vi "Properties_Insert Dotted Properties.vi"(11 "Property Info Array In":T1(array[cluster])) -> (1 "exe time (ms)":u32, 2 "Stop":bool, 3 "Property Info Array Out":T1(array[cluster]))   [LabVIEW 2023]
doc: "Find all dottable properties and insert dotted properties after them in list."
panel:
  out "dotted":i32
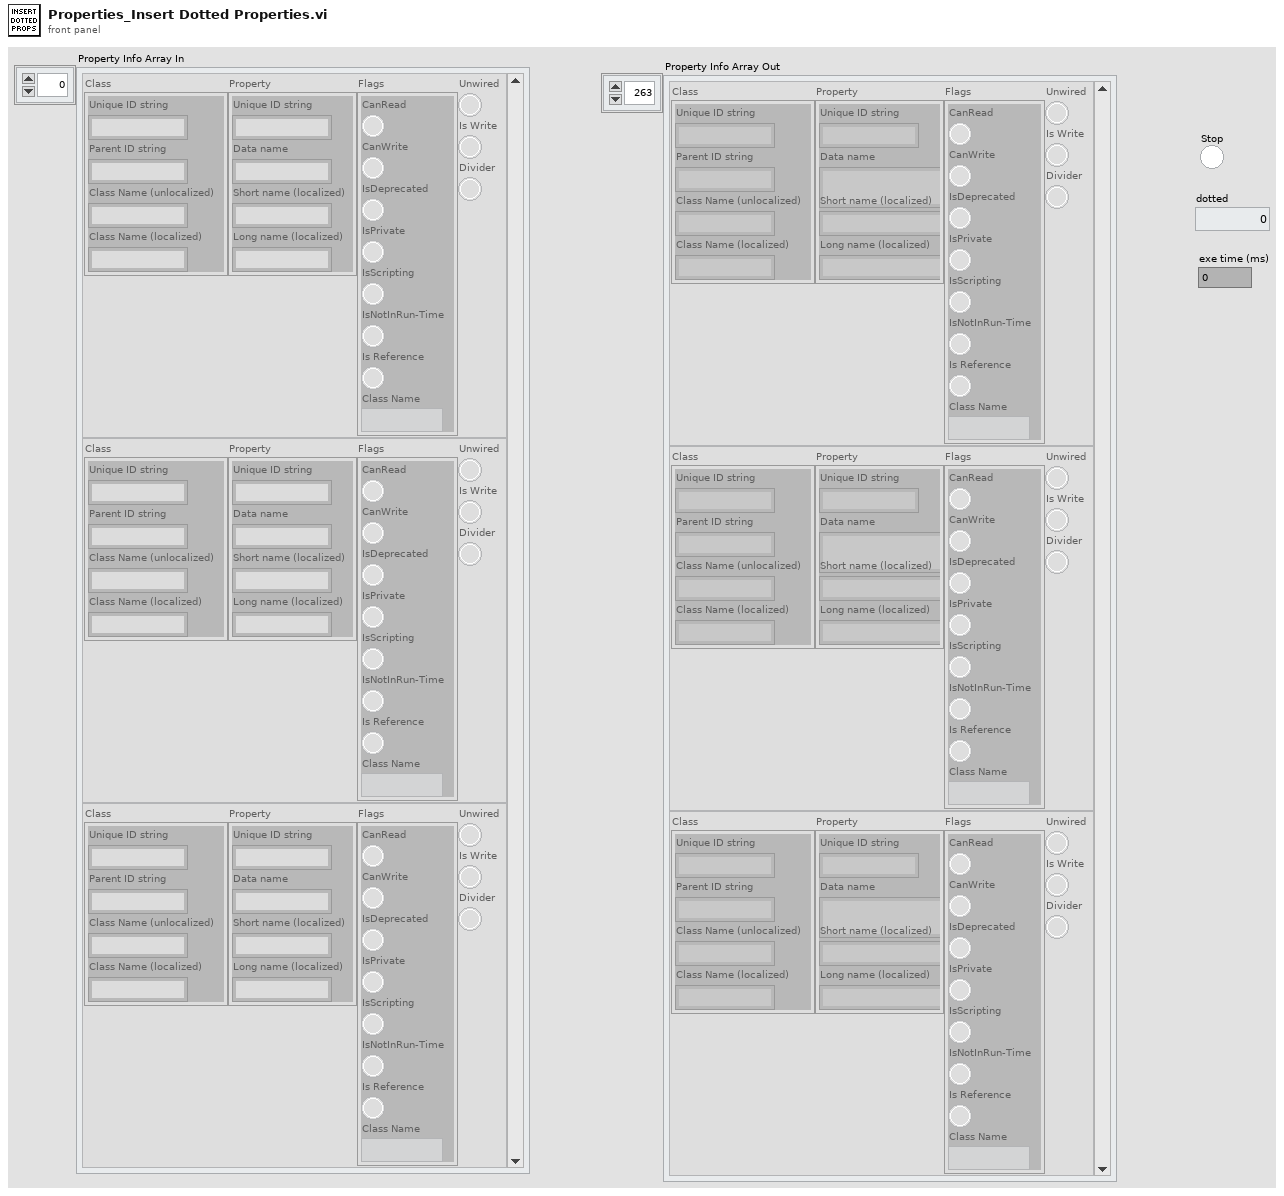
[diagram p1: front panel]
types:
  T1 = cluster{"Class":cluster{"Unique ID string":string, "Parent ID string":string, "Class Name (unlocalized)":string, "Class Name (localized)":string}, "Property":cluster{"Unique ID string":string, "Data name":string, "Short name (localized)":string, "Long name (localized)":string}, "Flags":cluster{"CanRead":bool, "CanWrite":bool, "IsDeprecated":bool, "IsPrivate":bool, "IsScripting":bool, "IsNotInRun-Time":bool, "Is Reference":bool, "Class Name":string}, "Divider":bool, "Is Write":bool, "Unwired":bool}[]
  T2 = cluster{"Class":cluster{"Unique ID string":string, "Parent ID string":string, "Class Name (unlocalized)":string, "Class Name (localized)":string}, "Property":cluster{"Unique ID string":string, "Data name":string, "Short name (localized)":string, "Long name (localized)":string}, "Flags":cluster{"CanRead":bool, "CanWrite":bool, "IsDeprecated":bool, "IsPrivate":bool, "IsScripting":bool, "IsNotInRun-Time":bool, "Is Reference":bool, "Class Name":string}, "Divider":bool, "Is Write":bool, "Unwired":bool}
  T3 = cluster{"Undotted Property":string, "Bare Property":string, "Is dotted?":bool, "Dot depth":i32, "Indent":i32, "Property Hierarchy":string[], "Parents":string[]}
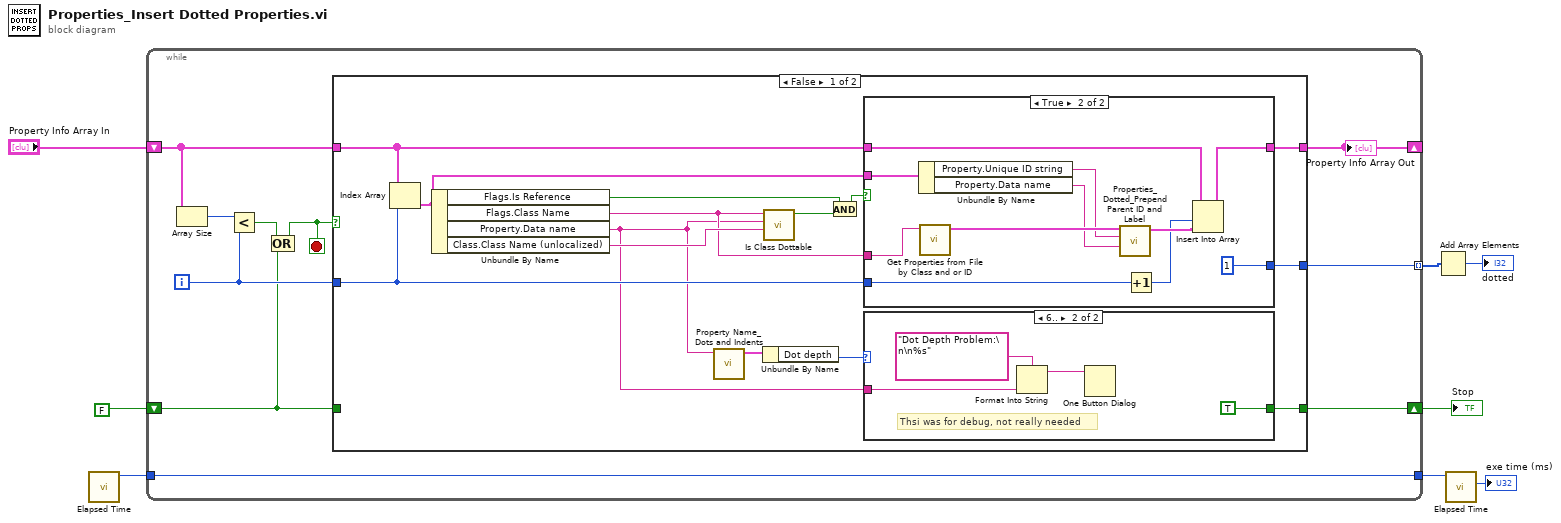
[diagram p0: block diagram]
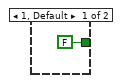
[diagram p2: hidden frame]
diagram:
  n1 = call "Elapsed Time.vi"() -> ("millisecond timer value"=w4:u32)  [unwired: 7 in, 4 out]
  n2 = while {
    shift-right: [w15] -> _
    shift-left: "Property Info Array In" -> [w18]
    shift-right: [w14] -> w6
    shift-left: FALSE -> [w11]
    tunnel: [w10] -> w5
    tunnel: w4 -> [w10]
    tunnel: [w9] -> w2 mode=indexing
    i -> [w16]
    stop <- w12 stop-if-true
    n3 = Array Size(array=w18) -> (size(s)=w17:i32)
    n4 = Less?(x=w17, y=w16) -> (x < y?=w13:bool)
    n5 = Compound Arithmetic op=OR(w13, w11) -> (w12:bool)
    n6 = case shown="False" w12 {
      tunnel: [w32 w51] -> w15
      tunnel: w18 -> [w31 w51]
      tunnel: w16 -> [w30 _]
      tunnel: [w23 w50] -> w14
      tunnel: w11 -> [_ w50]
      tunnel: [w21 _] -> w9
      frame False {
        n7 = Index Array(array=w31, index=w30) -> (element=w29:T2)
        n8 = Unbundle By Name(w29) -> ("Flags.Is Reference"=w26:bool, "Flags.Class Name"=w24:string, "Property.Data name"=w22:string, "Class.Class Name (unlocalized)"=w28:string)
        n9 = call "Property Name_Dots and Indents.vi"("Property"=w22) -> ("Cluster"=w20:T3)  [unwired: 10 in]
        n10 = Unbundle By Name(w20) -> ("Dot depth"=w19:i32)
        n11 = call "Is Class Dottable.vi"("Parent Class Name"=w28, "Property Name"=w22, "ClassName"=w24) -> ("Dottable"=w27:bool)  [unwired: 6 in, 2 out]
        n12 = And(x=w26, y=w27) -> (x .and. y?=w25:bool)
        n13 = case shown="True" w25 {
          tunnel: [w38 w48] -> w32
          tunnel: w31 -> [w38 w47]
          tunnel: w30 -> [_ w49]
          tunnel: w29 -> [_ w43]
          tunnel: w24 -> [_ w40]
          tunnel: [_ 1] -> w21
          frame False {
          }
          frame True {
            n14 = Unbundle By Name(w43) -> ("Property.Unique ID string"=w42:string, "Property.Data name"=w41:string)
            n15 = call "Get Properties from File by Class and or ID.vi"("Class Name"=w40) -> ("Array"=w46:T1)  [unwired: 10 in]
            n16 = call "Properties_Dotted_Prepend Parent ID and Label.vi"("Parent Name"=w41, "Parent ID"=w42, "Property Arr In"=w46) -> ("Property Arr Out"=w45:T1)  [unwired: 8 in]
            n17 = Increment(x=w49) -> (x+1=w44:i32)
            n18 = Insert Into Array(array=w47, index=w44, new element=w45) -> (w48:T1)
          }
        }
        n19 = case shown="6.." w19 {
          tunnel: w22 -> [_ w36]
          tunnel: [FALSE TRUE] -> w23
          frame 1, Default {
          }
          frame 6.. {
            # "Thsi was for debug, not really needed"
            n20 = Format Into String(format string="Dot Depth Problem:\n\n%s", w36) -> (resulting string=w35:string)  [unwired: 2 in, 1 out]
            n21 = One Button Dialog(message=w35) -> ()  [unwired: 1 in, 1 out]
          }
        }
      }
      frame True {
      }
    }
    "Property Info Array Out" <- w15
  }
  "Stop" <- w6
  n22 = Add Array Elements(numeric array=w2) -> (sum=→"dotted":i32)
  n23 = call "Elapsed Time.vi"("past time"=w5) -> ("elapsed time (ms)"=→"exe time (ms)":u32)  [unwired: 6 in, 4 out]
